vi "Power Spectral Density Estimation.vi"() -> ()   [LabVIEW 2023]
doc: "This example demonstrates how to estimate the power spectrum density (PSD) of a univariate time series by using different methods. This example uses the TSA Periodogram VI, the TSA Welch VI, the TSA Capon Spectrum VI, the TSA AR Spectrum VI, and the TSA ARMA Spectrum to estimate the PSDs.\n\n<b>Instructions:</b>\n1) Run this VI.\n2) Compare the power spectral density (PSD) by using different PSD-estimation methods."
uses:
  <vilib>/addons/Time Series Analysis/Correlation and Spectral Analysis.llb/TSA ARMA Spectrum (Array).vi
  <vilib>/addons/Time Series Analysis/Correlation and Spectral Analysis.llb/TSA Periodogram (Array).vi
  <vilib>/addons/Time Series Analysis/Correlation and Spectral Analysis.llb/TSA AR Spectrum (Array).vi
  <vilib>/addons/Time Series Analysis/Correlation and Spectral Analysis.llb/TSA Welch (Array).vi
  <vilib>/addons/Time Series Analysis/Correlation and Spectral Analysis.llb/TSA Capon Spectrum (Real).vi
  <vilib>/Analysis/NI_AALBase.lvlib
  <vilib>/addons/_Advanced Signal Processing/NI_AdvSigProcTSA.lvlib
panel:
  in  "view 5":bool=TRUE
  in  "view 4":bool=TRUE
  in  "view 3":bool=TRUE
  in  "view 2":bool=TRUE
  in  "view":bool=TRUE
  in  "FIR filter length":i32=64
  in  "stop":bool
  in  "Window info":T1={"Window 2"=2, "Length"=128, "Overlap (%)"=90.0} {"Window 2" items=["None ", "Hanning", "Hamming", "Blackman-Harris", "Exact Blackman", "Blackman", "Flat Top", "4 Term B-Harris ", "7 Term B-Harris", "Low Sidelobe"]}
  in  "ARMA order":cluster{"AR":i32, "MA":i32}={"AR"=40, "MA"=6}
  in  "Method 2":u16(ring) items=["Yule-Walker", "High order AR", "Polynomial"]
  in  "AR order":i32=40
  in  "Method 1":u16(ring)=1 items=["Forward-Backward", "Least-Squares", "Yule-Walker", "Burg-Lattice", "Geometric-Lattice"]
  in  "Window":u16(ring)=1 items=["None ", "Hanning", "Hamming", "Blackman-Harris", "Exact Blackman", "Blackman", "Flat Top", "4 Term B-Harris ", "7 Term B-Harris", "Low Sidelobe"]
  in  "dB on? (T)":bool=TRUE
  in  "Frequency bins":i32=1024
  out "Power Spectral Density":cluster{"f0":dbl, "df":dbl, "S(f)":dbl[]}[](graph)
  # "Overview: Demonstrates how to estimate the power spectrum density (PSD) of a univariate time series by using different methods.\nInstructions: \n1. Run this VI.\n2. Compare the power spectral density (PSD) by using different PSD-estimation methods.\n3. Click Stop to stop the VI."
  # "Periodogram"
  # "Welch"
  # "Capon Spectrum"
  # "AR Spectrum"
  # "ARMA Spectrum"
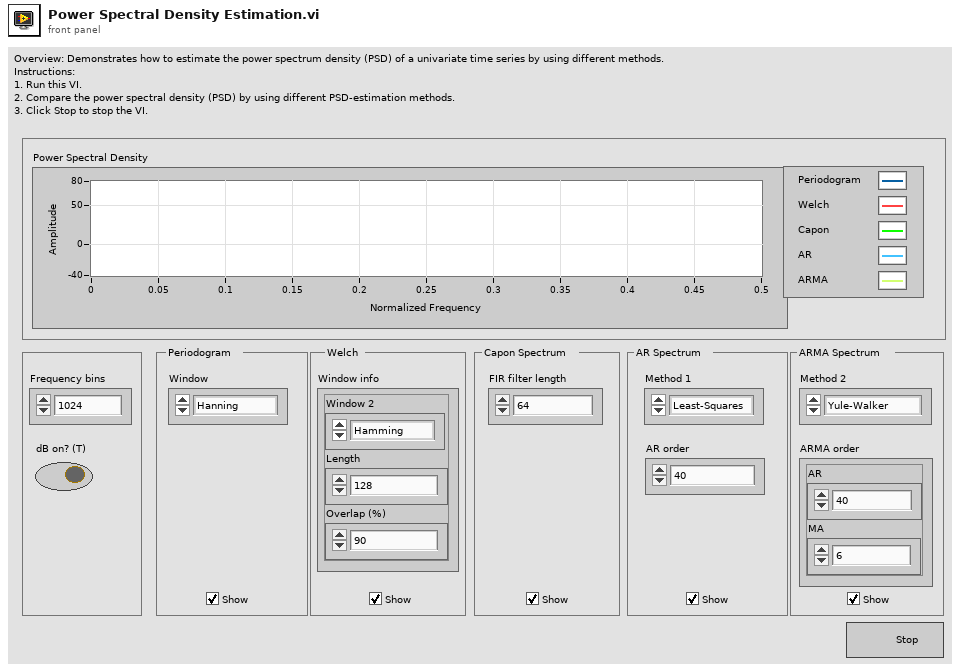
[diagram p1: front panel]
types:
  T1 = cluster{"Window 2":u16, "Length":i32, "Overlap (%)":dbl}
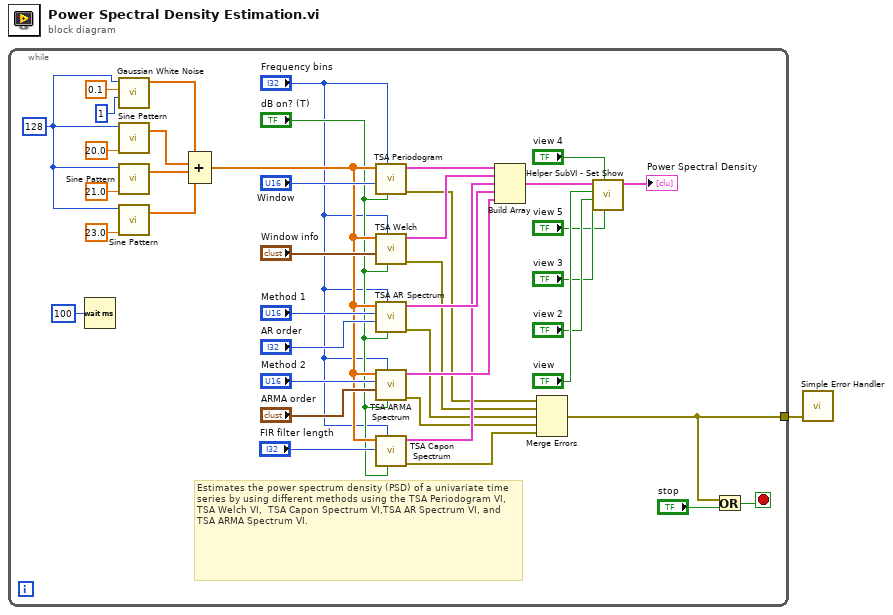
[diagram p0: block diagram]
diagram:
  n1 = while {
    tunnel: [w4] -> w1
    stop <- w2 stop-if-true
    w37 = 128 ("samples")
    # "Estimates the power spectrum density (PSD) of a univariate time series by using different methods using the TSA Periodogram VI, TSA Welch VI,  TSA Capon Spectrum VI,TSA AR Spectrum VI, and TSA ARMA Spectrum VI."
    n2 = Wait (ms)(milliseconds to wait=u32 100 ("millisecond multiple")) -> ()  [unwired: 1 out]
    n3 = call <vilib>:"Gaussian White Noise.vi"("seed"=1, "standard deviation"=0.1, "samples"=w37) -> ("Gaussian noise pattern"=w41:dbl[])  [unwired: 7 in, 1 out]
    n4 = call <vilib>:"Sine Pattern.vi"("cycles"=20.0, "samples"=w37) -> ("Sinusoidal Pattern"=w31:dbl[])  [unwired: 2 in, 1 out]
    n5 = call <vilib>:"Sine Pattern.vi"("cycles"=21.0, "samples"=w37) -> ("Sinusoidal Pattern"=w30:dbl[])  [unwired: 2 in, 1 out]
    n6 = call <vilib>:"Sine Pattern.vi"("cycles"=23.0, "samples"=w37) -> ("Sinusoidal Pattern"=w38:dbl[])  [unwired: 2 in, 1 out]
    n7 = Compound Arithmetic op=ADD(w41, w31, w30, w38) -> (w14:dbl[])
    n8 = call-poly <vilib>:"TSA Periodogram.vi"("dB on? (T)"="dB on? (T)", "frequency bins"="Frequency bins", "window"="Window", "Xt"=w14) -> ("error out"=w9:errorcluster, "PSD"=w36:cluster{"f0":dbl, "df":dbl, "S(f)":dbl[]})  [unwired: 1 in, 5 out]
    n9 = call-poly <vilib>:"TSA Welch.vi"("dB on? (T)"="dB on? (T)", "frequency bins"="Frequency bins", "window info"="Window info", "Xt"=w14) -> ("error out"=w8:errorcluster, "PSD"=w35:cluster{"f0":dbl, "df":dbl, "S(f)":dbl[]})  [unwired: 1 in, 5 out]
    n10 = call-poly <vilib>:"TSA AR Spectrum.vi"("dB on? (T)"="dB on? (T)", "frequency bins"="Frequency bins", "AR order"="AR order", "AR method"="Method 1", "Xt"=w14) -> ("error out"=w7:errorcluster, "PSD"=w23:cluster{"f0":dbl, "df":dbl, "S(f)":dbl[]})  [unwired: 1 in, 4 out]
    n11 = call-poly <vilib>:"TSA ARMA Spectrum.vi"("dB on? (T)"="dB on? (T)", "frequency bins"="Frequency bins", "ARMA order"="ARMA order", "method"="Method 2", "Xt"=w14) -> ("error out"=w6:errorcluster, "PSD"=w22:cluster{"f0":dbl, "df":dbl, "S(f)":dbl[]})  [unwired: 1 in, 4 out]
    n12 = call-poly <vilib>:"TSA Capon Spectrum.vi"("dB on? (T)"="dB on? (T)", "frequency bins"="Frequency bins", "FIR filter length"="FIR filter length", "Xt"=w14) -> ("error out"=w5:errorcluster, "PSD"=w10:cluster{"f0":dbl, "df":dbl, "S(f)":dbl[]})  [unwired: 2 in, 4 out]
    n13 = Build Array(w36, w35, w10, w23, w22) -> (w20:cluster{"f0":dbl, "df":dbl, "S(f)":dbl[]}[])
    n14 = Merge Errors(w9, w8, w7, w6, w5) -> (w4:errorcluster)
    n15 = call "Helper SubVI - Set Show.vi"("view 5"="view 5", "view 4"="view 4", "view 3"="view 3", "view 2"="view 2", "view"="view", "in"=w20) -> ("out"=→"Power Spectral Density":cluster{"f0":dbl, "df":dbl, "S(f)":dbl[]}[])  [unwired: 5 out]
    n16 = Or(x=w4, y="stop") -> (x .or. y?=w2:bool)
  }
  n17 = call <vilib>:"Simple Error Handler.vi"("error in (no error)"=w1) -> ()  [unwired: 4 in, 5 out]
